vi "PLC_OP20_Read.vi"(8 "error in (no error)":errorcluster, 11 "S7 Connection in":T1) -> (0 "error out":errorcluster, 3 "S7 Connection out 2":T1)   [LabVIEW 2017]
uses:
  <vilib>/DATA AHEAD/SP7/typedefs/S7 Connection.ctl
  <vilib>/DATA AHEAD/SP7/typedefs/PLC Type.ctl
  <vilib>/DATA AHEAD/SP7/functions/read/read real array.vi
  <vilib>/DATA AHEAD/SP7/functions/read/read String.vi
  <vilib>/DATA AHEAD/SP7/functions/read/read Dint array.vi
  <vilib>/DATA AHEAD/SP7/SP7.lvlib
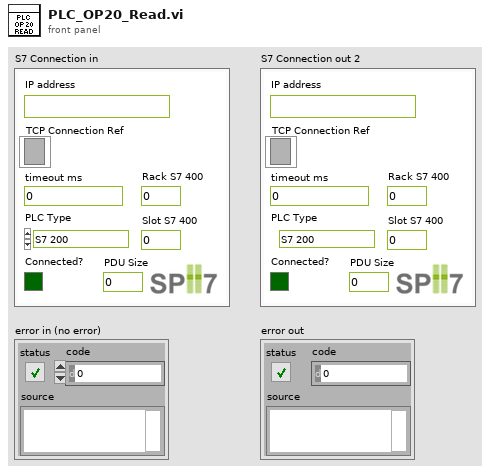
[diagram p1: front panel]
types:
  T1 = typedef "SP7.lvlib/S7 Connection.ctl" = cluster{"TCP Connection Ref":refnum<k5>, "IP address":string, "timeout ms":i32, "Connected?":bool, "PLC Type":T2, "Rack S7 400":u8, "Slot S7 400":u8, "PDU Size":u16, "connection semaphore":T3}
  T2 = typedef "SP7.lvlib/PLC Type.ctl" = enum16{"S7 200", "S7 300/400", "S7 1200", "S7 1500", "LOGO!8"}
  T3 = typedef "Semaphore RefNum" = refnum<k1>
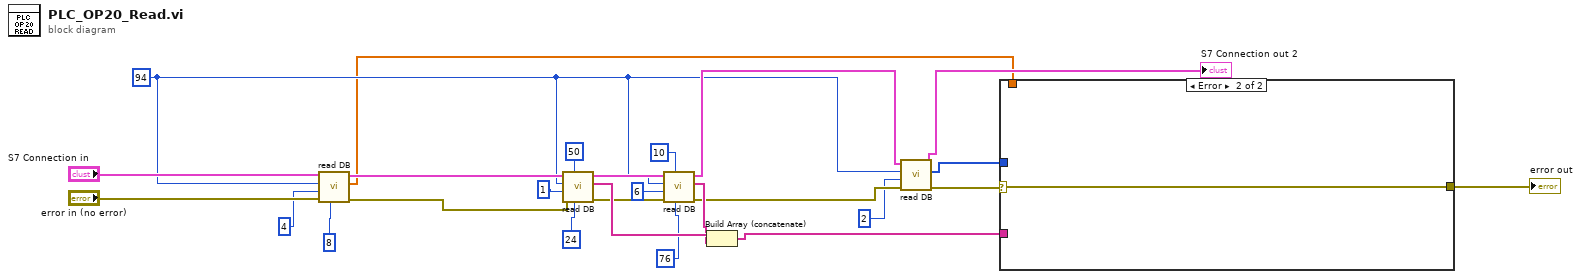
[diagram p0: block diagram]
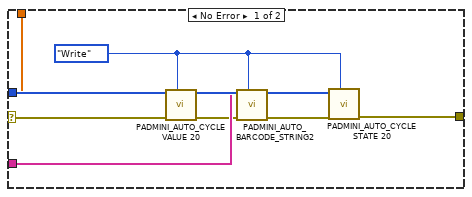
[diagram p2: hidden frame]
diagram:
  w4 = u16 94 ("Data Block #")
  n1 = call-poly <vilib>:"read DB.vi"("Item offset [byte]"=u32 8, "error in (no error)"="error in (no error)", "items #"=u16 4 ("Items # [byte]"), "Data Block #"=w4, "S7 Connection in"="S7 Connection in") -> ("error out"=w10:errorcluster, "REAL result array"=w1:sgl[], "S7 Connection out"=w14:T1)  [unwired: 4 in]
  n2 = call-poly <vilib>:"read DB.vi"("Item offset [byte]"=u32 24, "String length reserved in DB (default=254)"=u32 50 ("Item offset [byte]"), "error in (no error)"=w10, "items #"=u16 1 ("Items # [byte]"), "Data Block #"=w4, "S7 Connection in"=w14) -> ("error out"=w17:errorcluster, "STRING result Array"=w24:string[], "S7 Connection out"=w19:T1)  [unwired: 2 in, 1 out]
  n3 = call-poly <vilib>:"read DB.vi"("Item offset [byte]"=u32 76, "String length reserved in DB (default=254)"=u32 10 ("Item offset [byte]"), "error in (no error)"=w17, "items #"=u16 6 ("Items # [byte]"), "Data Block #"=w4, "S7 Connection in"=w19) -> ("error out"=w18:errorcluster, "STRING result Array"=w23:string[], "S7 Connection out"=w6:T1)  [unwired: 2 in, 1 out]
  n4 = Build Array (concatenate)(w24, w23) -> (w2:string[])
  n5 = call-poly <vilib>:"read DB.vi"("error in (no error)"=w18, "items #"=u16 2 ("Items # [byte]"), "Data Block #"=w4, "S7 Connection in"=w6) -> ("error out"=w7:errorcluster, "DINT result array"=w9:i32[], "S7 Connection out"=→"S7 Connection out 2":T1)  [unwired: 5 in]
  n6 = case shown="Error" w7 {
    selector: w7 -> [w29 w35]
    tunnel: w9 -> [w34 _]
    tunnel: [w33 w35] -> w3
    tunnel: w2 -> [w31 _]
    tunnel: w1 -> [w27 _]
    frame No Error {
      w28 = enum16{"Read", "Write"}."Write" ("Enum")
      n7 = call "PADMINI_AUTO_CYCLE VALUE 20.vi"("Enum"=w28, "error in (no error)"=w29, "Input"=w27) -> ("error out"=w30:errorcluster)  [unwired: 7 in, 1 out]
      n8 = call "PADMINI_AUTO_BARCODE_STRING2.vi"("Enum"=w28, "error in (no error)"=w30, "Input"=w31) -> ("error out"=w32:errorcluster)  [unwired: 7 in, 1 out]
      n9 = call "PADMINI_AUTO_CYCLE STATE 20.vi"("Enum"=w28, "error in (no error)"=w32, "Input"=w34) -> ("error out"=w33:errorcluster)  [unwired: 7 in, 1 out]
    }
    frame Error {
    }
  }
  "error out" <- w3
